vi "Recurse.vi"(6 "Error":errorcluster, 7 "BaseActor":refnum<class "BaseActor.lvclass">, 11 "Message":refnum<class "Message.lvclass">) -> (3 "Message":refnum<class "Message.lvclass">, 4 "Error":errorcluster, 5 "BaseActor":refnum<class "BaseActor.lvclass">)   [LabVIEW 2020, in "jettl.lvlib" / "BaseActor.lvlib" / "BaseActor.lvclass"]
uses:
  BaseActor.lvclass
  BaseActor.lvclass/BaseActor.ctl
  Message/Message.lvclass
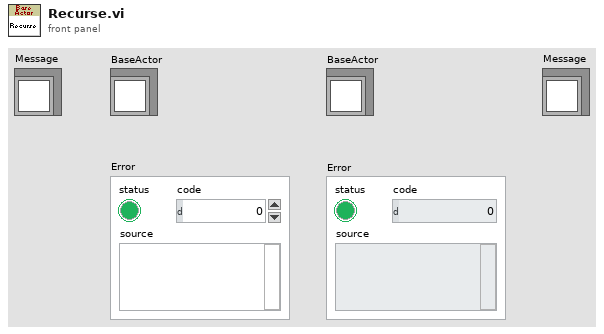
[diagram p1: front panel]
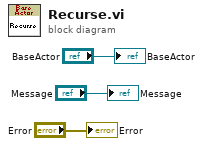
[diagram p0: block diagram]
diagram:
  "BaseActor" <- "BaseActor"
  "Error" <- "Error"
  "Message" <- "Message"
